vi "Digital Pulse Generate_RPM.vi"() -> ()   [LabVIEW 2019, in "Part of Main VIs.lvlib"]
uses:
  Part of Main VIs.lvlib
  <vilib>/Utility/error.llb/DialogType.ctl
  <vilib>/DAQmx/read.llb/DAQmx Read (Analog 1D DBL 1Chan NSamp).vi
  <extravilib>/ChannelInstances/Tag-a[.](dbl)/Read With Abort.vi
  <extravilib>/ChannelInstances/Tag-a[.](dbl)/Write With Abort.vi
  <extravilib>/ChannelInstances/Tag-dbl/Write With Abort.vi
  <extravilib>/ChannelInstances/Tag-dbl/Read With Abort.vi
  <vilib>/DAQmx/create/channels.llb/DAQmx Create Channel (CO-Pulse Generation-Time).vi
  <vilib>/DAQmx/configure/timing.llb/DAQmx Timing (Implicit).vi
  <extravilib>/ChannelInstances/Tag-dbl/Instantiate.vi
  <extravilib>/ChannelInstances/Tag-dbl/EndpointRead.vi
  <extravilib>/ChannelInstances/Tag-dbl/Endpoint.vi
  <vilib>/DAQmx/create/channels.llb/DAQmx Create Channel (AI-Voltage-Basic).vi
  <vilib>/DAQmx/configure/timing.llb/DAQmx Timing (Sample Clock).vi
  <vilib>/DAQmx/miscellaneous.llb/DAQmx Fill In Error Info.vi
  <extravilib>/ChannelInstances/Tag-a[.](dbl)/Instantiate.vi
  <extravilib>/ChannelInstances/Tag-a[.](dbl)/EndpointRead.vi
  <extravilib>/ChannelInstances/Tag-a[.](dbl)/Endpoint.vi
  <resource>/objmgr/daqmx.rc
  <extravilib>/ChannelInstances/Tag-dbl.lvlib
  SubVIs.lvlib
  <extravilib>/ChannelInstances/Tag-a[.](dbl).lvlib
panel:
  out "SampClk.Timebase.Src":tag
  out "SampClk.Src":tag
  out "Amplitude Chart":dbl[](graph)
  out "Amplitude Graph":waveform(dbl)(graph)
  out "RPM":dbl(knob) scale=0.0..1260.0
  out "Pulses":dbl[](array[numeric]) format="%0.2f"
  out "Pulse per sec":dbl[](array[numeric])
  out "RPM Array":dbl[](array[numeric])
  out "Pulse per 100ms":dbl[](array[numeric])
  out "Low Time":dbl
  in  "RPM":dbl=1000.0
  out "Period":dbl
  out "Frequency":dbl
  out "CO.CtrTimebaseSrc":tag
  out "CO.Pulse.Term":tag
  out "CO.Pulse.HighTime":dbl
  out "CO.Pulse.LowTime":dbl
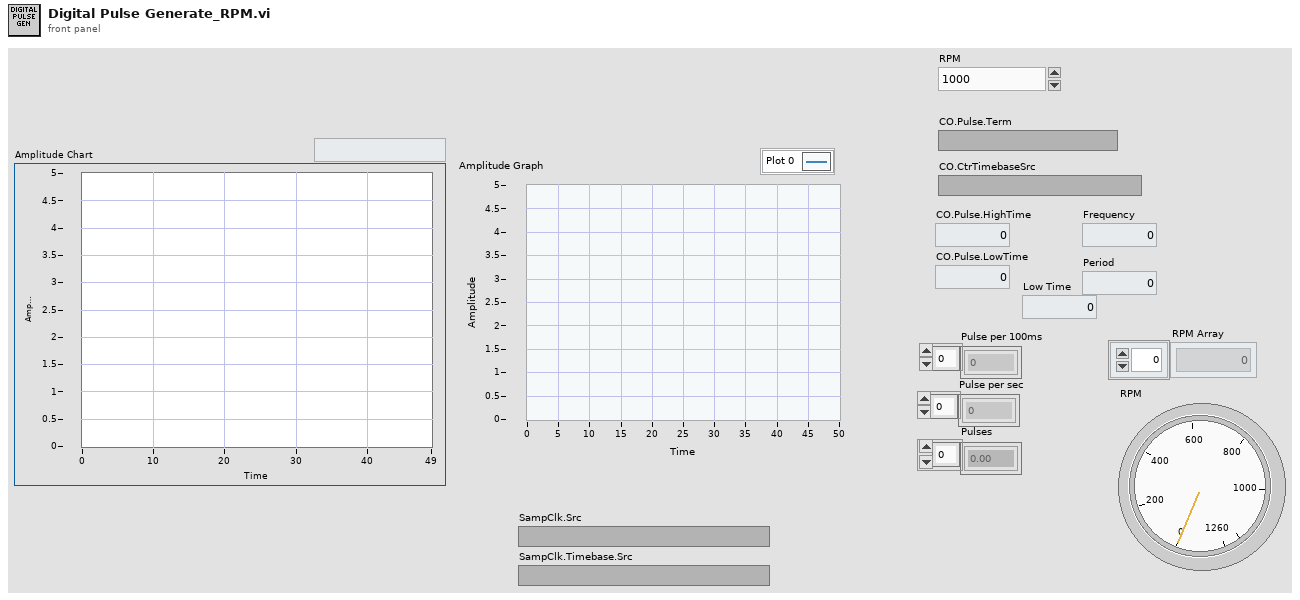
[diagram p1: front panel]
types:
  T1 = typedef "DialogType.ctl" = u16
  T2 = typedef "Tag-dbl.lvlib/))Channel.ctl" = refnum<queue>
  T3 = typedef "Tag-a[.](dbl).lvlib/))Channel.ctl" = refnum<queue>
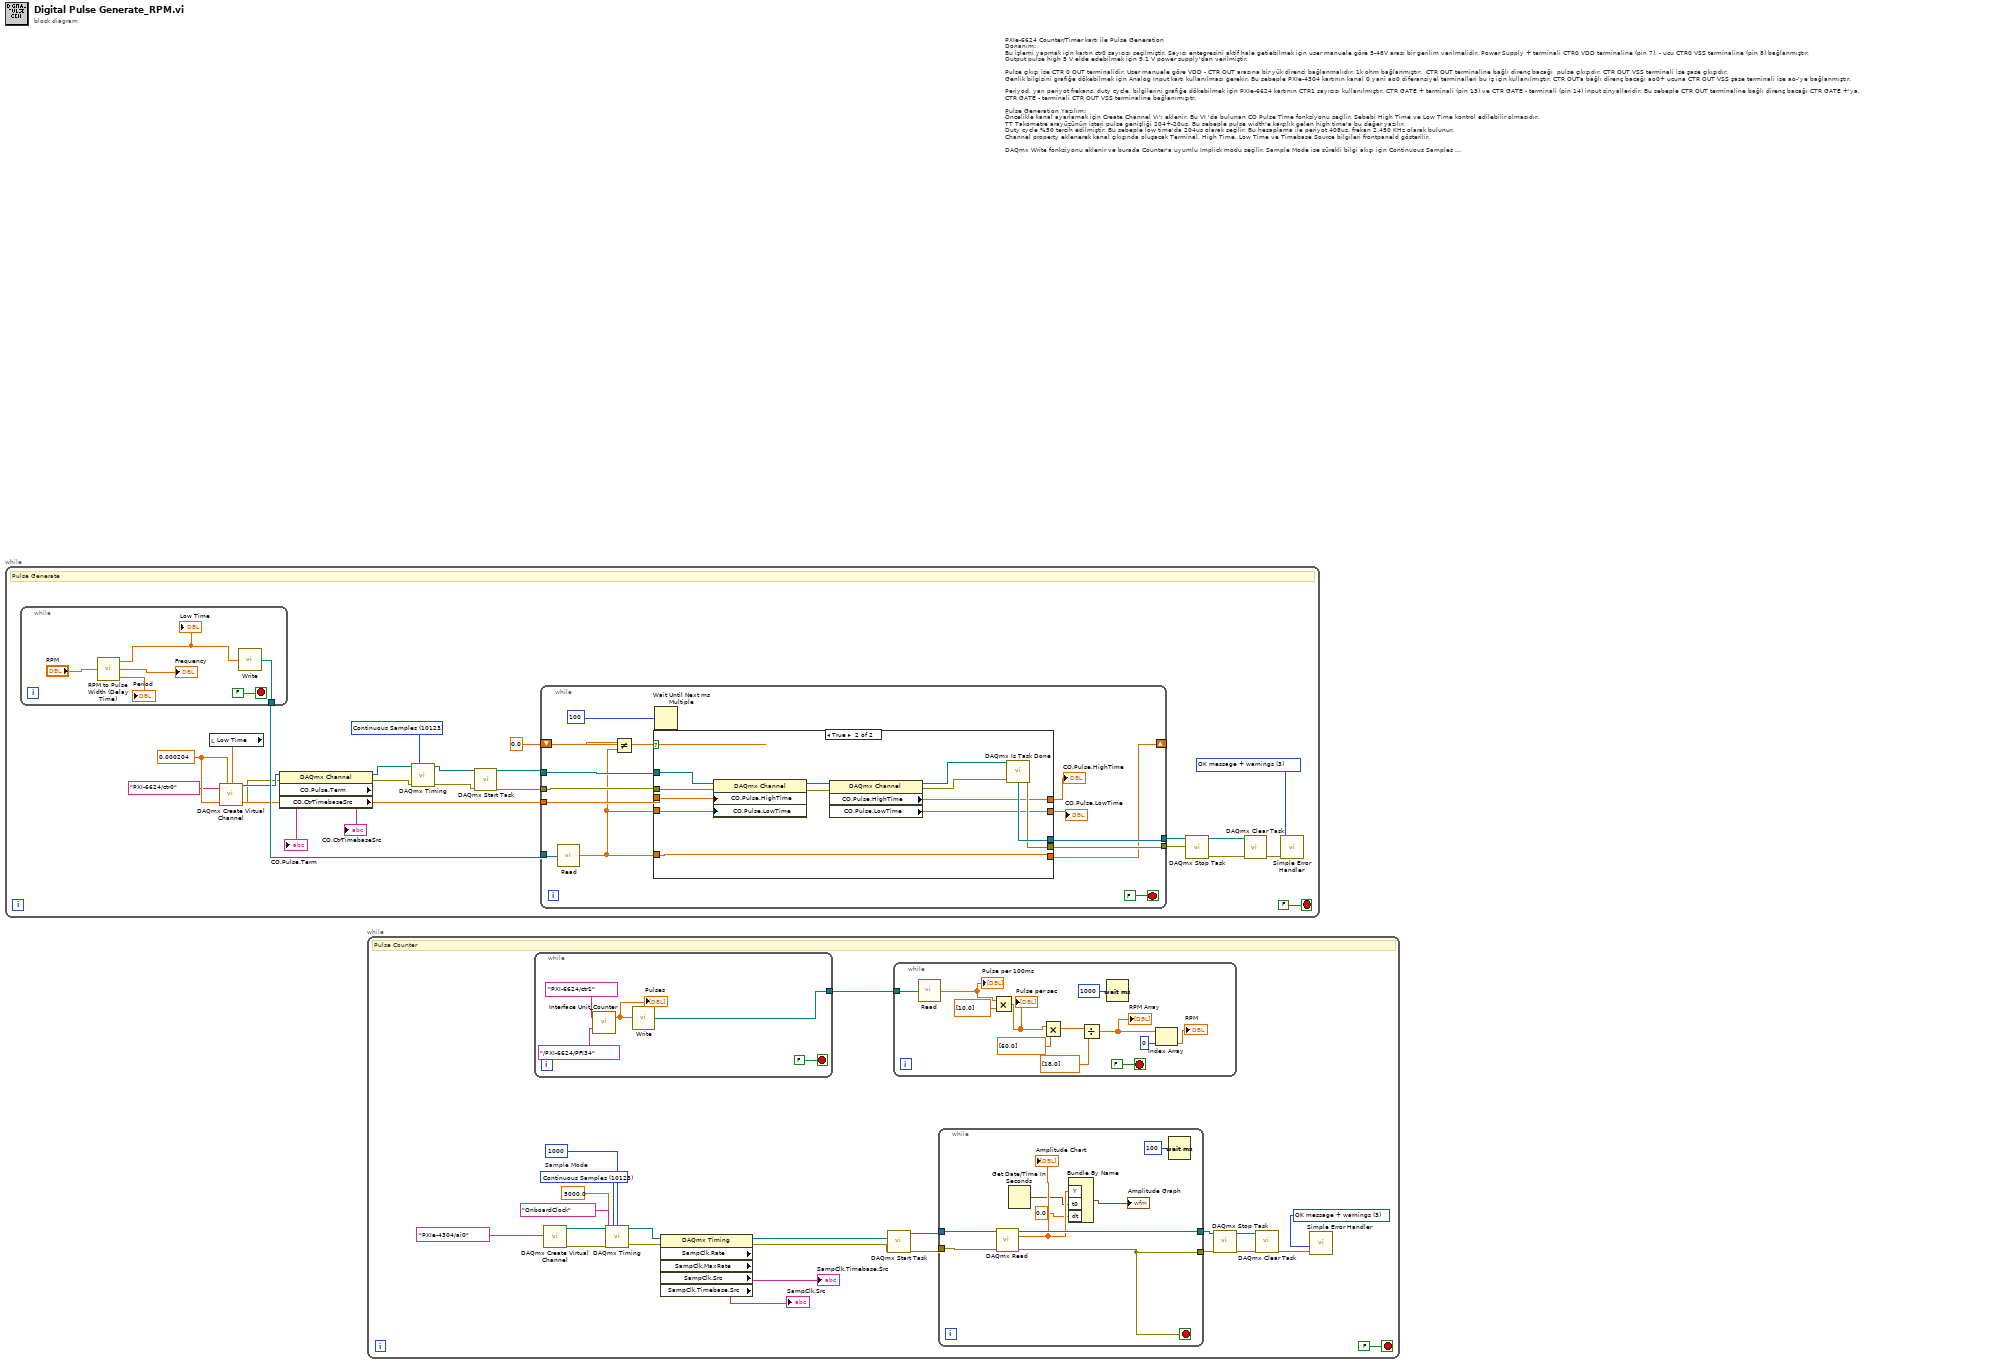
[diagram p0: block diagram]
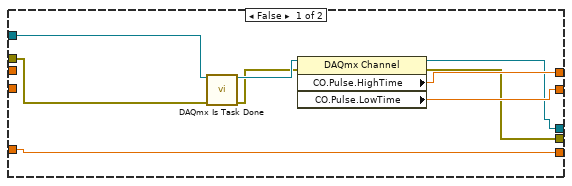
[diagram p2: hidden frame]
diagram:
  # "PXIe-6624 Counter/Timer kartı ile Pulse Generation\nDonanım:\nBu işlemi yapmak için kartın ctr0 sayıcısı seçilmiştir. Sayıcı entegresini aktif hale getiebilmek için user manuele göre 5-48V arası bir gerilim verilmelidir. Power Supply + terminali CTR0 VDD terminaline (pin 7), - ucu CTR0 VSS terminaline (pin 8) bağlanmıştır. \nOutput pulse high 5 V elde edebilmek için 9.1 V power supply'dan verilmiştir. \n\nPulse çıkışı ise CTR 0 OUT terminalidir. User manuele göre VDD - CTR OUT arasına bir yük direnci bağlanmalıdır. 1k ohm bağlanmıştır.  CTR OUT terminaline bağlı direnç bacağı  pulse çıkışıdır. CTR OUT VSS terminali ise şase çıkışıdır.\nGenlik bilgisini grafiğe dökebilmek için Analog Input kartı kullanılması gerekir. Bu sebeple PXIe-4304 kartının kanal 0 yani ao0 diferansiyel terminalleri bu iş için kullanılmıştır. CTR OUTa bağlı direnç bacağı ao0+ ucuna CTR OUT VSS şase terminali ise ao-'ye bağlanmıştır.\n\nPeriyod, yarı periyot frekans, duty cycle, bilgilerini grafiğe dökebilmek için PXIe-6624 kartının CTR1 sayıcısı kullanılmıştır. CTR GATE + terminali (pin 13) ve CTR GATE - terminali (pin 14) input sinyalleridir. Bu sebeple CTR OUT terminaline bağlı direnç bacağı CTR GATE +'ya,\nCTR GATE - terminali CTR OUT VSS terminaline bağlanımışıtr. \n\nPulse Generation Yazılım:\nÖncelikle kanal ayarlamak için Create Channel Vı'ı eklenir. Bu VI 'da bulunan CO Pulse Time fonksiyonu seçilir. Sebebi High Time ve Low Time kontrol edilebilir olmasıdır. \nTT Takometre arayüzünün isteri pulse genişliği 204+-20us. Bu sebeple pulse width'e karşılık gelen high time'a bu değer yazılır. \nDuty cycle %50 tercih edilmiştir. Bu sebeple low time'da 204us olarak seçilir. Bu hesaplama ile periyot 408us, frekan 2.450 KHz olarak bulunur.\nChannel property eklenerek kanal çıkışında oluşacak Terminal, High Time, Low Time ve Timebase Source bilgileri frontpaneld gösterilir.\n\nDAQmx Write fonksiyonu eklenir ve burada Counter'a uyumlu Implick modu seçilir. Sample Mode ise sürekli bilgi akışı için Continuous Samples seçilir.\nGörevi başlatmak için Start VI'ı eklenir.\nStop btonuna basana kadar dönecek DAQmx is Task Done Vı'ı ile pulse üretimi gerçekleştirilir."
  n1 = while {
    stop <- FALSE stop-if-true
    w16 = 0.000204 ("high time")
    w15 = 10123 items=["Finite Samples"=10178, "Continuous Samples"=10123, "Hardware Timed Single Point"=12522] ("sample mode")
    w21 = T1 3 items=["no dialog", "OK message", "continue or stop message", "OK message + warnings", "continue/stop + warnings"] ("type of dialog (OK msg:1)")
    # "Pulse Generate"
    n2 = while {
      tunnel: [w64] -> w23
      stop <- FALSE stop-if-true
      n3 = call "RPM to Pulse Width (Delay Time).vi"("RPM"="RPM") -> ("Period"=→"Period":dbl, "Frequency"=→"Frequency":dbl, "Low Time"=w60:dbl)  [unwired: 2 in]
      "Low Time" <- w60
      n4 = call <extravilib>:"Write.vi"("element"=w60) -> ("channel"=w64:T2)  [unwired: 1 out]
    }
    n5 = local read "Low Time"() -> (w8:dbl)
    n6 = call-poly <vilib>:"DAQmx Create Virtual Channel.vi"("high time"=w16, "low time"=w8, "counter"=tag "PXI-6624/ctr0") -> ("task out"=w13:refnum<k21>, "error out"=w12:errorcluster)  [unwired: 11 in]
    n7 = property class="DAQmx Channel"(reference=w13, error in=w12) -> (reference out=w7:refnum<k21>, error out=w6:errorcluster, "CO.Pulse.Term"=→"CO.Pulse.Term":tag, "CO.CtrTimebaseSrc"=→"CO.CtrTimebaseSrc":tag)
    n8 = call-poly <vilib>:"DAQmx Timing.vi"("task/channels in"=w7, "sample mode"=w15, "error in"=w6) -> ("task out"=w5:refnum<k21>, "error out"=w4:errorcluster)  [unwired: 11 in]
    n9 = call <vilib>:"DAQmx Start Task.vi"("task/channels in"=w5, "error in"=w4) -> ("task out"=w3:refnum<k21>, "error out"=w2:errorcluster)  [unwired: 12 in]
    n10 = while {
      tunnel: w2 -> [w34]
      tunnel: w3 -> [w35]
      shift-right: [w28] -> _
      shift-left: 0.0 ("element") -> [w29]
      tunnel: w16 -> [w27]
      tunnel: [w33] -> w18
      tunnel: [w32] -> w17
      tunnel: w23 -> [w26]
      stop <- FALSE stop-if-true
      n11 = call <extravilib>:"Read.vi"("channel"=w26) -> ("element"=w25:dbl)  [unwired: 1 in, 1 out]
      n12 = Not Equal?(x=w29, y=w25) -> (x != y?=w36:bool)
      n13 = case shown="True" w36 {
        tunnel: w35 -> [w46 w59]
        tunnel: w34 -> [w45 w58]
        tunnel: w27 -> [_ w55]
        tunnel: [w40 w57] -> w33
        tunnel: [w39 w56] -> w32
        tunnel: [w42 w52] -> w31
        tunnel: [w41 w51] -> w30
        tunnel: w25 -> [w38 w47]
        tunnel: [w38 w47] -> w28
        tunnel: w25 -> [_ w48]
        frame False {
          n14 = call <vilib>:"DAQmx Is Task Done.vi"("task/channels in"=w46, "error in"=w45) -> ("task out"=w44:refnum<k21>, "error out"=w43:errorcluster)  [unwired: 11 in, 1 out]
          n15 = property class="DAQmx Channel"(reference=w44, error in=w43) -> (reference out=w40:refnum<k21>, error out=w39:errorcluster, "CO.Pulse.HighTime"=w42:dbl, "CO.Pulse.LowTime"=w41:dbl)
        }
        frame True {
          n16 = property class="DAQmx Channel"(reference=w59, error in=w58, "CO.Pulse.HighTime"=w55, "CO.Pulse.LowTime"=w48) -> (reference out=w54:refnum<k21>, error out=w53:errorcluster)
          n17 = property class="DAQmx Channel"(reference=w54, error in=w53) -> (reference out=w50:refnum<k21>, error out=w49:errorcluster, "CO.Pulse.HighTime"=w52:dbl, "CO.Pulse.LowTime"=w51:dbl)
          n18 = call <vilib>:"DAQmx Is Task Done.vi"("task/channels in"=w50, "error in"=w49) -> ("task out"=w57:refnum<k21>, "error out"=w56:errorcluster)  [unwired: 11 in, 1 out]
        }
      }
      "CO.Pulse.HighTime" <- w31
      "CO.Pulse.LowTime" <- w30
      n19 = Wait Until Next ms Multiple(millisecond multiple=100) -> ()  [unwired: 1 out]
    }
    n20 = call <vilib>:"DAQmx Stop Task.vi"("task/channels in"=w18, "error in"=w17) -> ("task out"=w20:refnum<k21>, "error out"=w19:errorcluster)  [unwired: 12 in]
    n21 = call <vilib>:"DAQmx Clear Task.vi"("task in"=w20, "error in"=w19) -> ("error out"=w22:errorcluster)  [unwired: 13 in]
    n22 = call <vilib>:"Simple Error Handler.vi"("type of dialog (OK msg:1)"=w21, "error in (no error)"=w22) -> ()  [unwired: 3 in, 5 out]
  }
  n23 = while {
    stop <- FALSE stop-if-true
    w81 = 10123 items=["Finite Samples"=10178, "Continuous Samples"=10123, "Hardware Timed Single Point"=12522]  # Sample Mode
    w87 = T1 3 items=["no dialog", "OK message", "continue or stop message", "OK message + warnings", "continue/stop + warnings"] ("type of dialog (OK msg:1)")
    # "Pulse Counter"
    n24 = while {
      tunnel: [w110] -> w88
      stop <- FALSE stop-if-true
      n25 = call "Interface Unit_Counter.vi"("CI.CountEdges.Term"=tag "/PXI-6624/PFI34", "Counter Physical Channel"=tag "PXI-6624/ctr1") -> ("data"=w111:dbl[])  [unwired: 1 out]
      "Pulses" <- w111
      n26 = call <extravilib>:"Write.vi"("element"=w111) -> ("channel"=w110:T3)  [unwired: 1 out]
    }
    n27 = call-poly <vilib>:"DAQmx Create Virtual Channel.vi"("physical channels"=tag "PXIe-4304/ai0") -> ("task out"=w79:refnum<k21>, "error out"=w80:errorcluster)  [unwired: 13 in]
    n28 = call-poly <vilib>:"DAQmx Timing.vi"("task/channels in"=w79, "sample mode"=w81, "samples per channel"=1000, "rate"=5000.0, "source"=tag "OnboardClock", "error in"=w80) -> ("task out"=w83:refnum<k21>, "error out"=w82:errorcluster)  [unwired: 8 in]
    n29 = property class="DAQmx Timing" props=["SampClk.Rate", "SampClk.MaxRate", "SampClk.Src", "SampClk.Timebase.Src"](reference=w83, error in=w82) -> (reference out=w75:refnum<k21>, error out=w74:errorcluster, "SampClk.Src"=→"SampClk.Src":tag, "SampClk.Timebase.Src"=→"SampClk.Timebase.Src":tag)  [unwired: 2 out]
    n30 = call <vilib>:"DAQmx Start Task.vi"("task/channels in"=w75, "error in"=w74) -> ("task out"=w71:refnum<k21>, "error out"=w70:errorcluster)  [unwired: 12 in]
    n31 = while {
      tunnel: w88 -> [w102]
      stop <- FALSE stop-if-true
      n32 = call <extravilib>:"Read.vi"("channel"=w102) -> ("element"=w101:dbl[])  [unwired: 1 in, 1 out]
      "Pulse per 100ms" <- w101
      n33 = Multiply(x=w101, y=dbl[] [10.0]) -> (x*y=w104:dbl[])
      "Pulse per sec" <- w104
      n34 = Multiply(x=w104, y=dbl[] [60.0]) -> (x*y=w107:dbl[])
      n35 = Divide(x=w107, y=dbl[] [18.0]) -> (x/y=w99:dbl[])
      "RPM Array" <- w99
      n36 = Wait (ms)(milliseconds to wait=u32 1000) -> ()  [unwired: 1 out]
      n37 = Index Array(array=w99, index=0) -> (element=→"RPM":dbl)
    }
    n38 = while {
      tunnel: w70 -> [w95]
      tunnel: [w89] -> w72
      tunnel: w71 -> [w96]
      tunnel: [w97] -> w73
      stop <- w89 stop-if-true
      n39 = call-poly <vilib>:"DAQmx Read.vi"("task/channels in"=w96, "error in"=w95) -> ("task out"=w97:refnum<k21>, "data"=w93:dbl[], "error out"=w89:errorcluster)  [unwired: 11 in]
      "Amplitude Chart" <- w93
      n40 = Get Date/Time In Seconds() -> (seconds since 1Jan1904=w92:timestamp)
      n41 = Bundle By Name("Y"=w93, "t0"=w92, "dt"=0.0) -> (→"Amplitude Graph":waveform(dbl))  [unwired: 1 in]
      n42 = Wait (ms)(milliseconds to wait=u32 100) -> ()  [unwired: 1 out]
    }
    n43 = call <vilib>:"DAQmx Stop Task.vi"("task/channels in"=w73, "error in"=w72) -> ("task out"=w86:refnum<k21>, "error out"=w85:errorcluster)  [unwired: 12 in]
    n44 = call <vilib>:"DAQmx Clear Task.vi"("task in"=w86, "error in"=w85) -> ("error out"=w84:errorcluster)  [unwired: 13 in]
    n45 = call <vilib>:"Simple Error Handler.vi"("type of dialog (OK msg:1)"=w87, "error in (no error)"=w84) -> ()  [unwired: 3 in, 5 out]
  }
